vi "Read NI 9475 - Digital Output.vi"(8 "error in":errorcluster, 11 "NI 9475 in":refnum<class "NI 9475.lvclass">) -> (0 "error out":errorcluster, 2 "channel settings":T1[](array[typedef]), 3 "NI 9475 out":refnum<class "NI 9475.lvclass">)   [LabVIEW 2017, in "Scan Engine Scripting.lvlib" / "NI 9475.lvclass"]
uses:
  NI 9475.lvclass
  Mode Classes/Controls/digital channel settings.ctl
  Scan Engine Scripting.lvlib
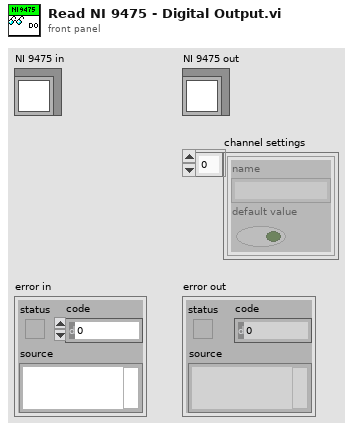
[diagram p1: front panel]
types:
  T1 = typedef "Scan Engine Scripting.lvlib/digital channel settings.ctl" = cluster{"name":string, "default value":bool}
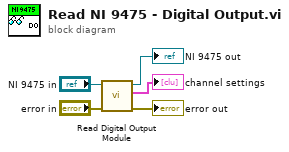
[diagram p0: block diagram]
diagram:
  n1 = call-dynamic "Read Digital Output Module.vi"("error in"="error in", "module in"="NI 9475 in") -> ("error out"=→"error out":errorcluster, "channel settings"=→"channel settings":T1[], "module out"=→"NI 9475 out":refnum<class "NI 9475.lvclass">)  [unwired: 7 in]
